vi "IntakeTeleop.vi"(8 "CmdCancel":bool, 9 "CmdFeedToShoot":bool, 10 "CmdSpitOut":bool, 11 "CmdIntake":bool) -> ()   [LabVIEW 2023]
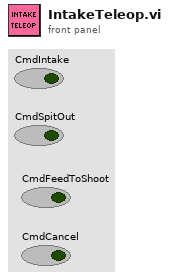
[diagram p1: front panel]
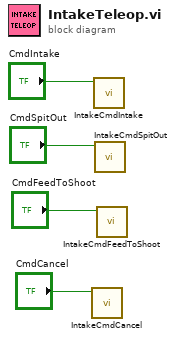
[diagram p0: block diagram]
diagram:
  n1 = call "IntakeCmdCancel.vi"("CmdCancel"="CmdCancel") -> ()  [unwired: 11 in]
  n2 = call "IntakeCmdIntake.vi"("CmdIntake"="CmdIntake") -> ()  [unwired: 11 in]
  n3 = call "IntakeCmdSpitOut.vi"("CmdSpitOut"="CmdSpitOut") -> ()  [unwired: 11 in]
  n4 = call "IntakeCmdFeedToShoot.vi"("CmdFeedToShoot"="CmdFeedToShoot") -> ()  [unwired: 11 in]
